vi "p_measure loop.vi"(7 "Calibration , nm":u32=275 min=220 max=1100 step=1) -> ()   [LabVIEW 2012]
doc: "This example VI for the Keithley 236 SMU allows the operator to select a source function, value and range. The VI\nputs the SMU in operate, sends a trigger and returns a single DC measurement. Also included in this VI are two error displays. Error out shows GPIB errors and device dependent errors shows errors generated by the machine."
uses:
  <vilib>/Analysis/NI_AALBase.lvlib
panel:
  in  "Average":i32
  out "Filter":string="\r\n"
  out "Range now":string="\r\n"
  out "Set auto":string="\r\n"
  out "Overrange":bool
  out "Power in nW":dbl format="%.6f"
  out "Read Wavelength":i32
  in  "error in (no error)":errorcluster
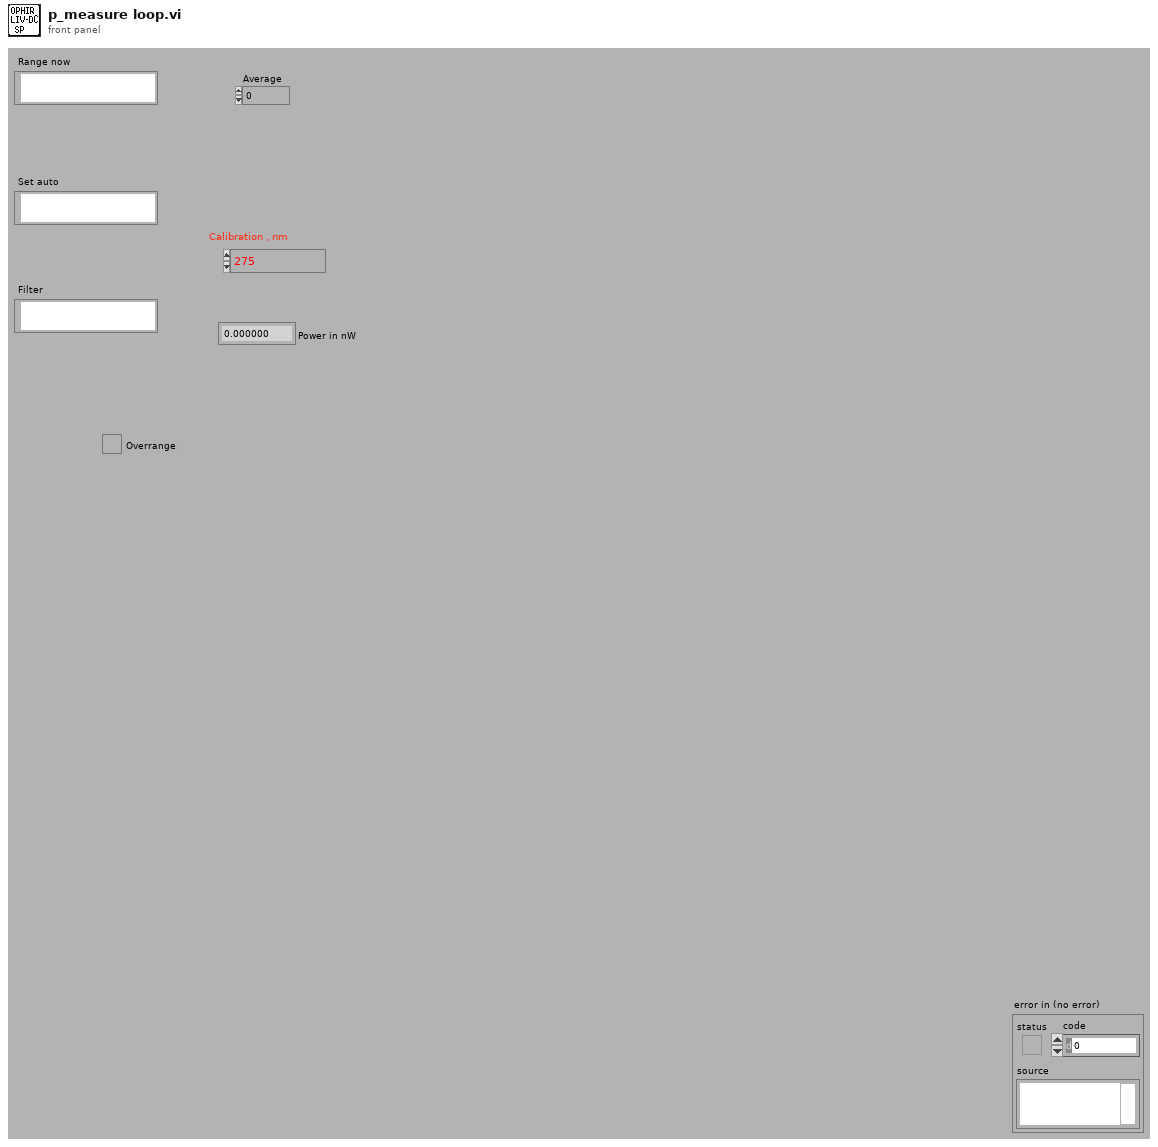
[diagram p1: front panel]
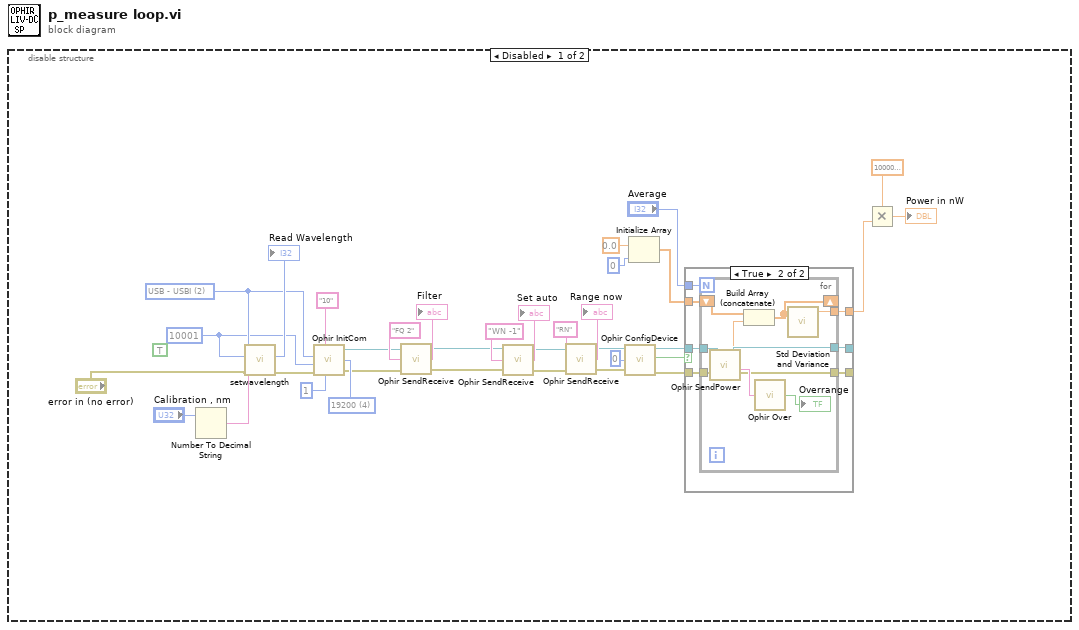
[diagram p0: block diagram]
diagram:
  n1 = disable-structure shown="Disabled" {
    frame Disabled {
      w25 = i16 4 items=["300", "1200", "4800", "9600", "19200", "38400"] ("Baud Rate (3:9600)")
      w10 = i16 10001 ("usb channel")
      w11 = u16 2 items=["USB - Nova2", "USB - Vega", "USB - USBI", "RS232", "GPIB"] ("Select Communication Protocol")
      (unwired) TRUE
      n2 = Number To Decimal String(number="Calibration , nm") -> (decimal integer string=w34:string)  [unwired: 1 in]
      n3 = call "setwavelength.vi"("error in (no error)"="error in (no error)", "Set Wavelength"=w34, "usb channel"=w10, "Select Communication Protocol"=w11) -> ("error out"=w9:errorcluster, "Read Wavelength"=→"Read Wavelength":i32)  [unwired: 6 in]
      n4 = call "Ophir InitCom.vi"("GPIB Address (10)"="10", "communication"=w11, "Numeric"=w10, "Port Number (default 2)"=i16 1, "error in (no error)"=w9, "Baud Rate (3:9600)"=w25) -> ("dup Visa Session"=w5:refnum<visa-resource-name>, "error out"=w3:errorcluster)  [unwired: 1 out]
      n5 = call "Ophir SendReceive.vi"("error in (no error)"=w3, "Command"="FQ 2", "Visa Session"=w5) -> ("error out"=w2:errorcluster, "Frame Output"=→"Filter":string, "dup Visa Session"=w4:refnum<visa-resource-name>)
      n6 = call "Ophir SendReceive.vi"("error in (no error)"=w2, "Command"="WN -1", "Visa Session"=w4) -> ("error out"=w14:errorcluster, "Frame Output"=→"Set auto":string, "dup Visa Session"=w16:refnum<visa-resource-name>)
      n7 = call "Ophir SendReceive.vi"("error in (no error)"=w14, "Command"="RN", "Visa Session"=w16) -> ("error out"=w13:errorcluster, "Frame Output"=→"Range now":string, "dup Visa Session"=w15:refnum<visa-resource-name>)
      n8 = call "Ophir ConfigDevice.vi"("Visa Session"=w15, "Measure Choice (0:Power)"=u16 0, "error in (no error)"=w13) -> ("dup Visa Session"=w28:refnum<visa-resource-name>, "OK ?"=w29:bool, "error out"=w27:errorcluster)  [unwired: 1 out]
      n9 = Initialize Array(0.0 ("element"), 0 ("dimension size")) -> (w21:dbl[])
      n10 = case shown="True" w29 {
        tunnel: w28 -> [w36 w44]
        tunnel: w27 -> [w37 w43]
        tunnel: [w36 w42] -> _
        tunnel: [w37 w41] -> _
        tunnel: w21 -> [_ w40]
        tunnel: [_ w39] -> w12
        tunnel: "Average" -> [_ w38]
        frame False {
          # "Force Power Configuration failed"
        }
        frame True {
          n11 = for {
            N: w38 -> [_]
            tunnel: w44 -> [w54]
            tunnel: w43 -> [w53]
            tunnel: [w52] -> w42
            tunnel: [w49] -> w41
            shift-right: [w46] -> _
            shift-left: w40 -> [w48]
            tunnel: [w45] -> w39
            n12 = call "Ophir SendPower.vi"("Visa Session"=w54, "error in (no error)"=w53) -> ("dup Visa Session"=w52:refnum<visa-resource-name>, "Value Number"=w47:dbl, "Value String"=w51:string, "error out"=w49:errorcluster)
            n13 = Build Array (concatenate)(w48, w47) -> (w46:dbl[])
            n14 = call "Ophir Over.vi"("Value String"=w51) -> ("Overrange"=→"Overrange":bool)
            n15 = call <vilib>:"Std Deviation and Variance.vi"("X"=w46) -> ("mean"=w45:dbl)  [unwired: 1 in, 2 out]
          }
        }
      }
      n16 = Multiply(x=1000000.0, y=w12) -> (x*y=→"Power in nW":dbl)
    }
    frame Enabled {
    }
  }
